vi "Hardware-DI-B Pump Ref Setup-Host.vi"() -> ()   [LabVIEW 2016]
panel:
  in  "RefPumpVoltageOffset":sgl
  in  "RefPumpVoltageMultiplier":sgl
  in  "RefPumpCurrentOffset":sgl
  in  "RefPumpCurrentMultiplier":sgl
  in  "RefPumpTimeAxisOffset":sgl
  in  "RefPumpTimeAxisMultiplier":sgl
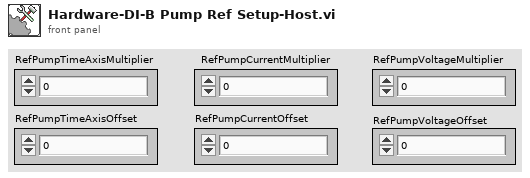
[diagram p1: front panel]
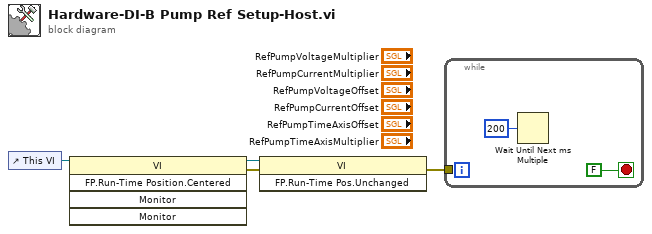
[diagram p0: block diagram]
diagram:
  n1 = control-ref of="This VI"() -> (w4:refnum<vi>)
  n2 = invoke class="VI" method="FP.Run-Time Position.Centered"(reference=w4) -> (reference out=w3:refnum<vi>, error out=w2:errorcluster)  [unwired: 4 in, 3 out]
  n3 = invoke class="VI" method="FP.Run-Time Pos.Unchanged"(reference=w3, error in=w2) -> (error out=w1:errorcluster)  [unwired: 1 in, 2 out]
  n4 = while {
    tunnel: w1 -> [_]
    stop <- FALSE stop-if-true
    n5 = Wait Until Next ms Multiple(millisecond multiple=u32 200) -> ()  [unwired: 1 out]
  }
